vi "Check Instance.vi"(8 "error in (no error)":errorcluster, 11 "PrefsDB in":refnum<class "PrefsDB.lvclass">) -> (0 "error out":errorcluster, 3 "PrefsDB out":refnum<class "PrefsDB.lvclass">)   [LabVIEW 2020, in "User Prefs.lvlib" / "PrefsDB.lvclass"]
uses:
  PrefsDB.lvclass
  PrefsDB.lvclass/PrefsDB.ctl
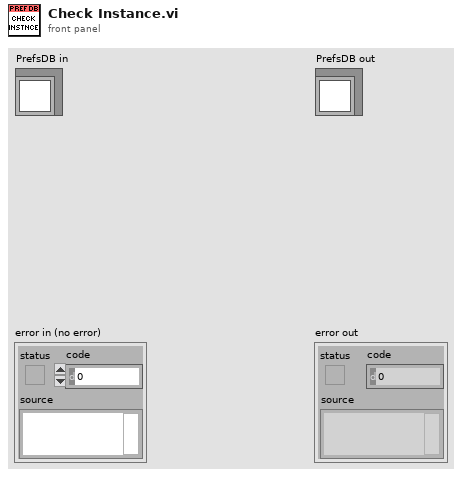
[diagram p1: front panel]
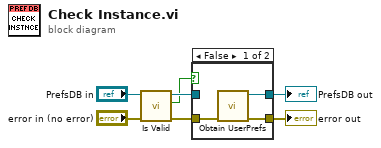
[diagram p0: block diagram]
diagram:
  n1 = call "Is Valid.vi"("error in (no error)"="error in (no error)", "PrefsDB in"="PrefsDB in") -> ("error out"=w7:errorcluster, "Is Valid"=w5:bool, "PrefsDB out"=w6:refnum<class "PrefsDB.lvclass">)  [unwired: 7 in]
  n2 = case shown="False" w5 {
    tunnel: w7 -> [w10 w11]
    tunnel: [w9 w11] -> w2
    tunnel: [w8 w12] -> w1
    tunnel: w6 -> [_ w12]
    frame False {
      n3 = call "Obtain UserPrefs.vi"("error in (no error)"=w10) -> ("error out"=w9:errorcluster, "PrefsDB out"=w8:refnum<class "PrefsDB.lvclass">)  [unwired: 9 in]
    }
    frame True {
    }
  }
  "error out" <- w2
  "PrefsDB out" <- w1
